vi "HitrapGUI.HTLE_TR6-LowerPart.vi"() -> ()   [LabVIEW 2014, in "HitrapGUI.lvlib"]
uses:
  HitrapGUI.lvlib
  CSlibraries/GUILib/GUILib.userEventsMainType.ctl
  CSlibraries-extern/DimLVEvent/DimIndicators/DimIndicators.anyType.ctl
  CSlibraries/GUILib/GUILib.simpleNumeric.ctl
  CSlibraries/GUILib/GUILib.basicNumeric.ctl
  CSlibraries-extern/DimLVEvent/DimIndicators/DimIndicators.numericType.ctl
  CSlibraries/UtilityLib/UtilityLib.valueStatus.ctl
  CSCore/CSSystem/CoreDefs/CoreDefs.rawDataType.ctl
  CSCore/CSSystem/CoreLib/CoreLib.double 2 byte array.vi
  CSCore/CSSystem/CoreLib/CoreLib.int 2 byte array.vi
  CSlibraries/UtilityLib/UtilityLib.lvlib
  CSCore/CSSystem/CSSystemLib/CSSystemLib.lvlib
  CSlibraries-extern/DimLVEvent/DimIndicators/DimIndicators.lvlib
  CSCore/GUIs/GOGControllerGUI/GOGControllerGUI.lvlib
  CSlibraries/GUILib/GUILib.lvlib
  CSCore/CSSystem/CoreLib/CoreLib.lvlib
  CSlibraries-extern/DimLVEvent/LVDimInterface/LVDimInterface.lvlib
panel:
  in  "TR6DK3Link":T1
  in  "MotorActivityLink-Act":T2
  in  "TR6QD3_2Ctl":T3 caption="TR6QD3_2" {"nom" step=1.0}
  in  "TR6QD3_1Ctl":T3 caption="TR6QD3_1" {"nom" step=1.0}
  in  "TR6DK3Ctl":T5 caption="TR6DK3" {"Progress Slide" scale=0.0..100.0; "Nom_Position" items=["Undefined", "Open", "Faraday Cup", "MCP"]}
  in  "userEventsMain 2":T6
  in  "userEventsMain":T6
  in  "MotorLink-Act":T2
  in  "TR6DK2Link":T1
  in  "TR6DK1Link":T1
  in  "TR6DK1Ctl":T5 caption="TR6DK1" {"Progress Slide" scale=0.0..100.0; "Nom_Position" items=["Undefined", "Open", "Faraday Cup", "MCP"]}
  in  "TR6DK2Ctl":T5 caption="TR6DK2" {"Progress Slide" scale=0.0..100.0; "Nom_Position" items=["Undefined", "Open", "Faraday Cup", "MCP"]}
  in  "Next":bool
  in  "Previous":bool
  in  "TR6QT1_3Ctl":T3 caption="TR6QT1_3" {"nom" step=1.0}
  in  "TR6QT1_2Ctl":T3 caption="TR6QT1_2" {"nom" step=1.0}
  in  "TR6KY3Ctl":T3 caption="TR6KY3" {"nom" step=1.0}
  in  "TR6DS2Ctl":T3 {"nom" step=1.0}
  in  "TR6KX3Ctl":T3 caption="TR6KX3" {"nom" step=1.0}
  in  "TR6QT1_1Ctl":T3 caption="TR6QT1_1" {"nom" step=1.0}
  in  "TR6QD2_2Ctl":T3 caption="TR6QD2_2" {"nom" step=1.0}
  in  "TR6QT1_3":bool=TRUE
  in  "TR6QT1_2":bool=TRUE
  in  "TR6QT1_1":bool=TRUE
  in  "TR6QD2_2":bool=TRUE
  in  "TR6KY3":bool=TRUE
  in  "TR6QD2_1Ctl":T3 caption="TR6QD2_1" {"nom" step=1.0}
  in  "TR6QD2_1":bool=TRUE
  in  "TR6DS2":bool=TRUE
  in  "TR5KX4":bool=TRUE
  in  "TR6MU1":bool=TRUE
  in  "TR6KY2":bool=TRUE
  in  "TR6KX2":bool=TRUE
  in  "TR6MU1Ctl":T3 caption="TR6MU1 - Field(mT)" {"nom" step=1.0}
  in  "TR6KY2Ctl":T3 caption="TR6KY2" {"nom" step=1.0}
  in  "TR6KX2Ctl":T3 caption="TR6KX2" {"nom" step=1.0}
  in  "TR6DS1":bool=TRUE
  in  "TR6DS1Ctl":T3 {"nom" step=1.0}
  in  "TR6QD1_2Ctl":T3 caption="TR6QD1_2" {"nom" step=1.0}
  in  "TR6QD1_1Ctl":T3 caption="TR6QD1_1" {"nom" step=1.0}
  in  "TR6QD1_2":bool=TRUE
  in  "TR6QD1_1":bool=TRUE
  in  "TR6KY1":bool=TRUE
  in  "TR6KY1Ctl":T3 caption="TR6KY1" {"nom" step=1.0}
  in  "TR6KX1Ctl":T3 caption="TR6KX1" {"nom" step=1.0}
  in  "TR6KX1":bool=TRUE
  in  "TR6ME1Ctl":T3 caption="TR6ME1" {"nom" step=1.0}
  in  "TR6ME1":bool=TRUE
  out "subSystem1State":string
  in  "subSystem1":bool
  out "subSystem1StateQuality":string
  in  "subControllersIgnoredDIM":T2
  in  "iniData":string
  in  "stop":bool
  in  "dummy":bool
  in  "parentSystem":bool
  in  "userEvent":refnum<user-event>
  # "TR6-LowerPart"
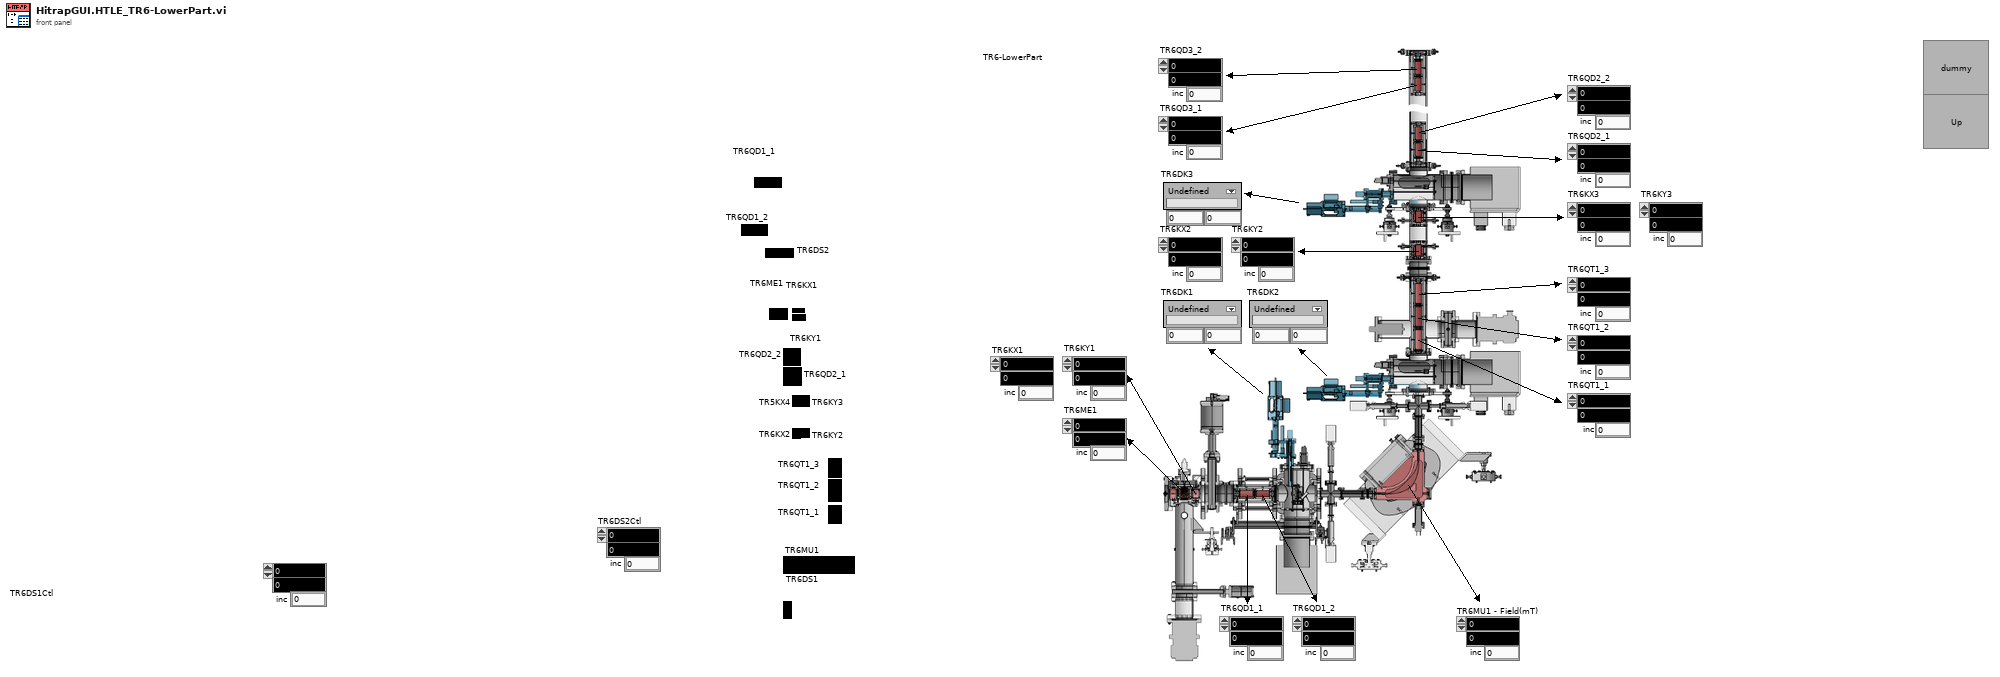
[diagram p1: front panel]
types:
  T1 = typedef "DimIndicators.lvlib/DimIndicators.numericType.ctl" = cluster{"data":dbl, "no link":bool, "quality":i32, "timeStamp":dbl}
  T2 = typedef "DimIndicators.lvlib/DimIndicators.anyType.ctl" = cluster{"data":string, "no link":bool, "quality":i32, "timeStamp":dbl}
  T3 = typedef "GUILib.lvlib/GUILib.simpleNumeric.ctl" = cluster{"nom":T4, "act":dbl, "inc":dbl}
  T4 = typedef "GUILib.lvlib/GUILib.basicNumeric.ctl" = dbl
  T5 = cluster{"Nom_Position":u8, "Progress Slide":u8, "TR6DK2Act":dbl, "TR6DK2Nom":dbl}
  T6 = typedef "GUILib.lvlib/GUILib.userEventsMainType.ctl" = cluster{"data":string, "dataType":i32}
  T7 = enum16{"Idle", "StartMotorActivity", "NewMotorDIM", "StopMotorActivity", "Stop"}
  T8 = typedef "UtilityLib.lvlib/UtilityLib.valueStatus.ctl" = enum16{"no info available", "stand by/off", "on", "warning", "alarm/malfunction", "not implemented", "user action required", "important information", "system default", "control default", "indicator default", "button default"}
  T9 = typedef "CoreDefs.rawDataType.ctl" = i8[]
  T10 = enum8{"Enabled", "Disabled", "Disabled and Grayed Out"}
  T11 = typedef "lveventtype.ctl" = enum32{"Null", "Timeout", "Annotation Menu Selection", "Annotation Menu Selection?", "App Instance Close", "App Instance Close?", "Autoscale Range Change", "Bookmark Info Change", "Cell Edit", "Cell Edit?", "Cursor Grab", "Cursor Grab?", "Cursor Menu Selection", "Cursor Menu Selection?", "Cursor Move", "Cursor Release", "Data Change", "Direction Change", "Display State Change", "Drag Ended", "Drag Enter", "Drag Leave", "Drag Over", "Drag Source Update", "Drag Starting", "Drag Starting?", "Drop", "Exec State Change", "Key Down", "Key Down?", "Key Repeat", "Key Repeat?", "Key Up", "Listbox Double Click", "Menu Activation?", "Menu Selection (App)", "Menu Selection? (App)", "Menu Selection (User)", "Mouse Down", "Mouse Down?", "Mouse Enter", "Mouse Leave", "Mouse Move", "Mouse Up", "Mouse Wheel", "NI Security User Change (App)", "Pane Size", "Panel Close", "Panel Close?", "Panel Resize", "Plot Attribute Change", "Scale Range Change", "Shortcut Menu Activation?", "Shortcut Menu Selection (App)", "Shortcut Menu Selection? (App)", "Shortcut Menu Selection (User)", "Tree Double Click", "Tree Drag", "Tree Drag?", "Tree Drop", "Tree Drop?", "Tree Item Close", "Tree Item Close?", "Tree Item Open", "Tree Item Open?", "User Event", "Value Change"}
  T12 = cluster{"TR6DK2Ctl":refnum<vi>, "byteArray out":T9}
  T13 = typedef "HitrapGUI.lvlib/HitrapGUI.i attribute.ctl" = cluster{"SVs":refnum<k21>[], "DSCIntProc":string, "MotorActivityID":i32}
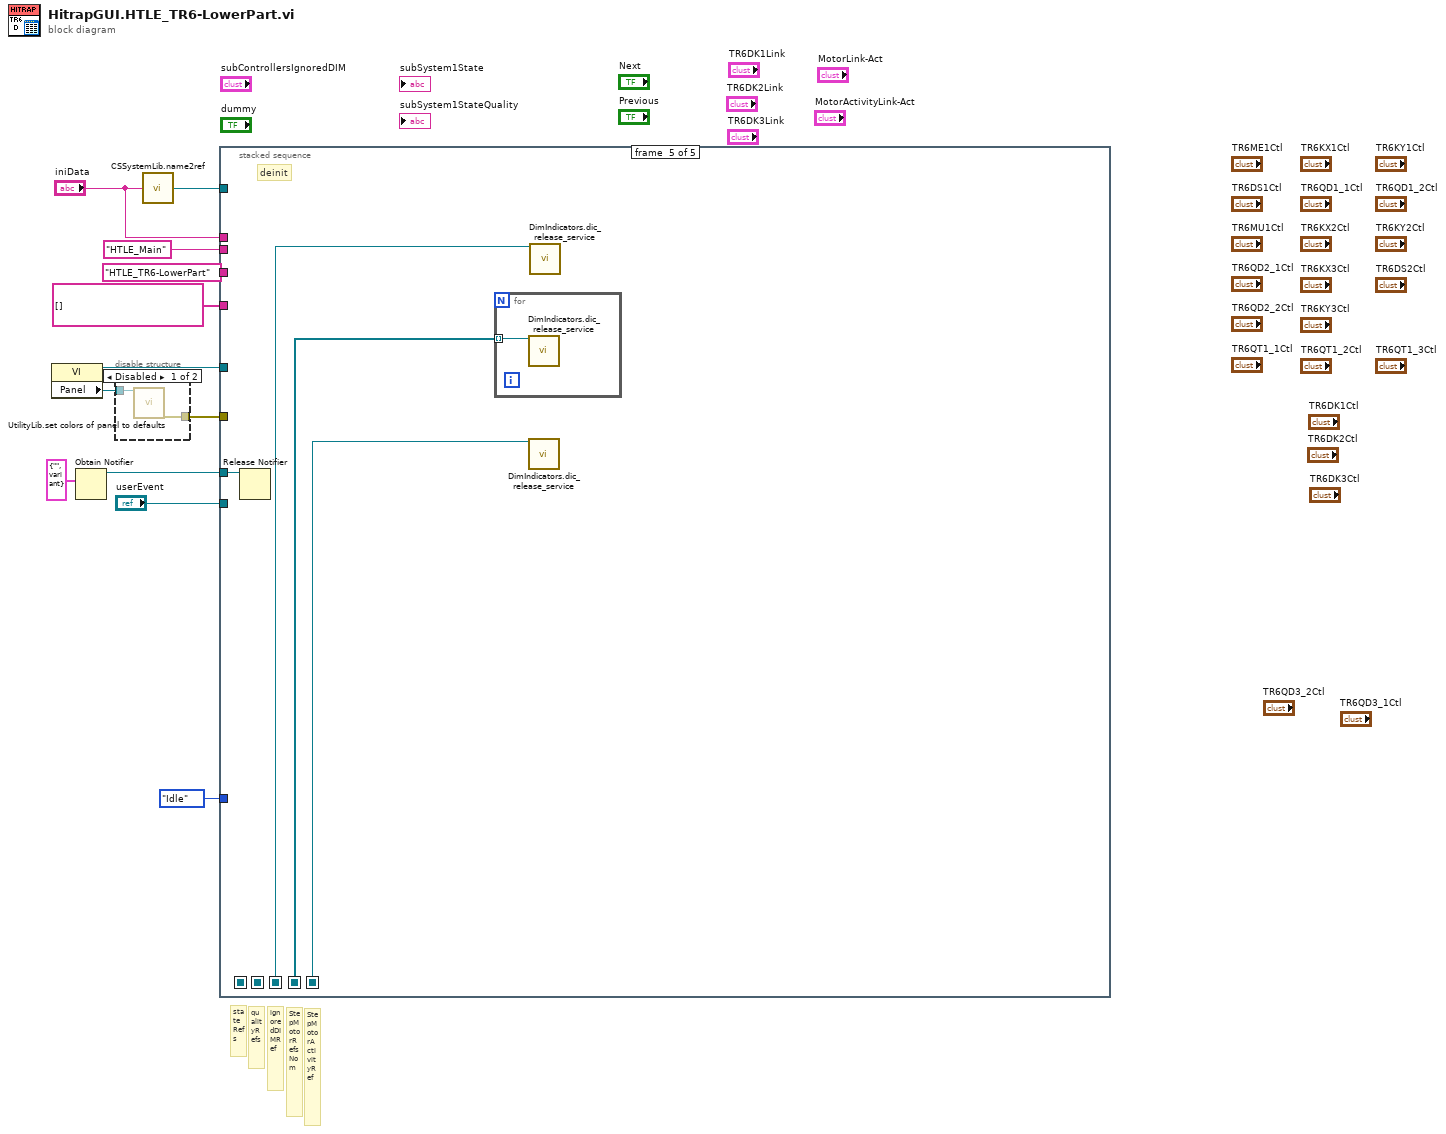
[diagram p0: block diagram]
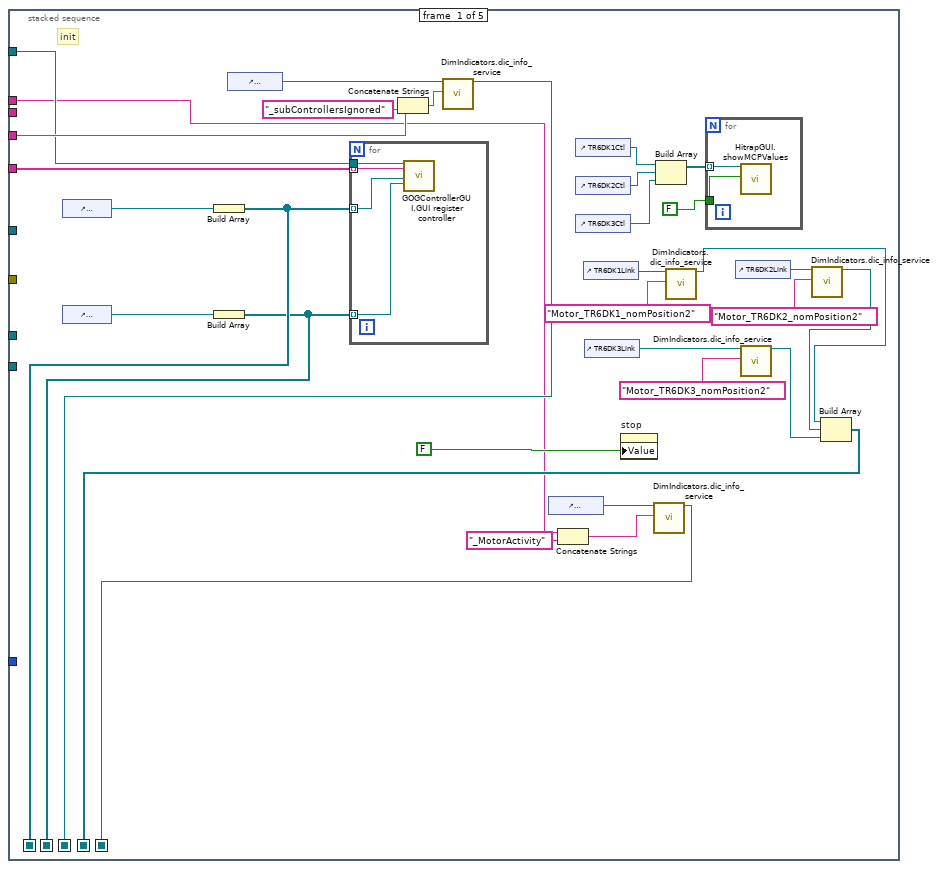
[diagram p3: hidden frame]
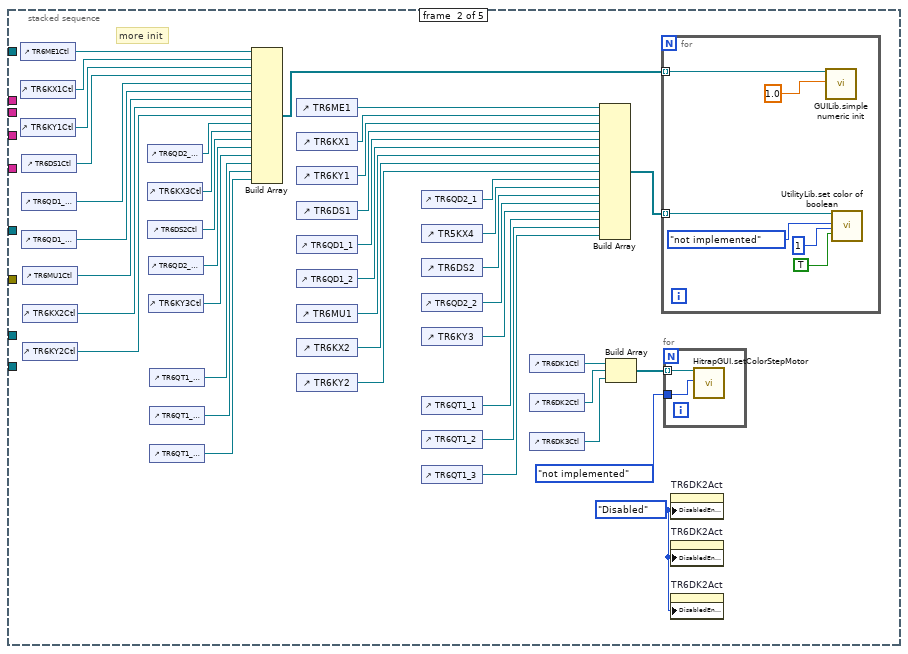
[diagram p4: hidden frame]
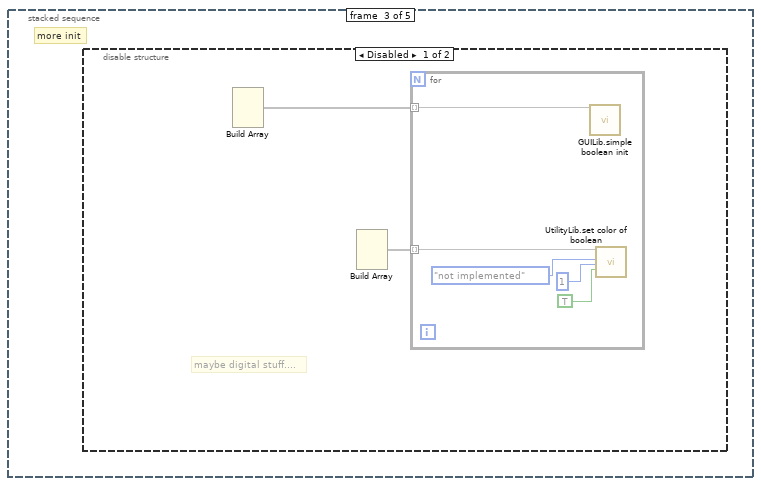
[diagram p5: hidden frame]
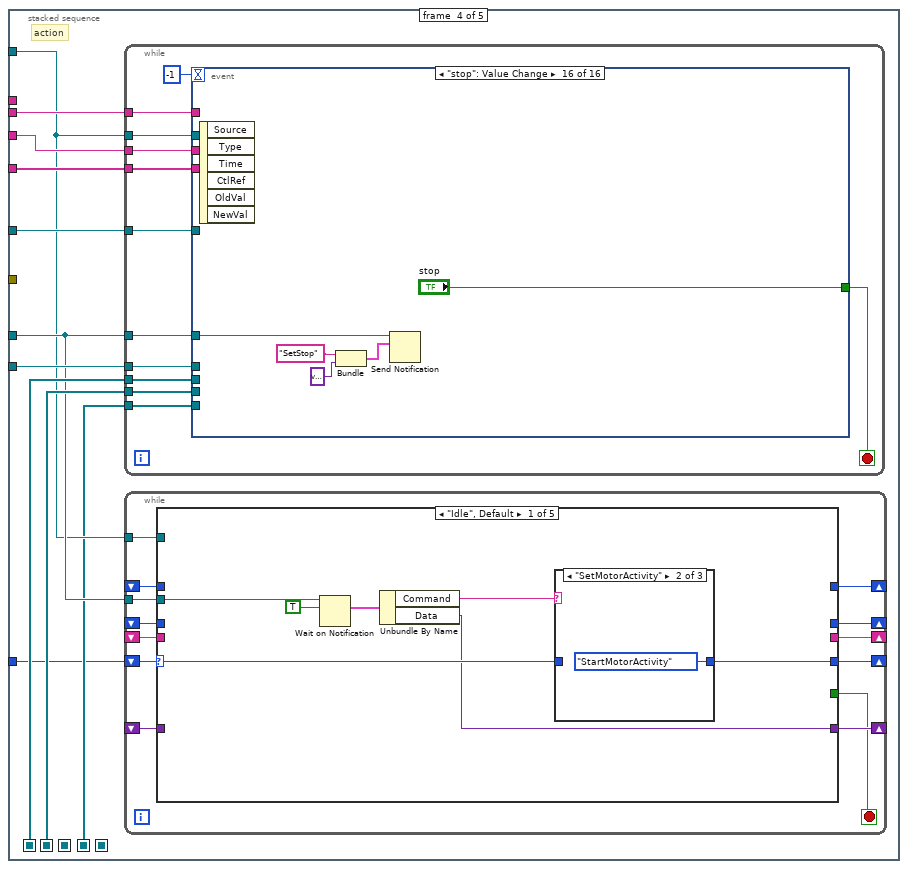
[diagram p7: hidden frame]
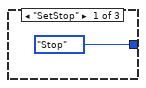
[diagram p8: hidden frame]
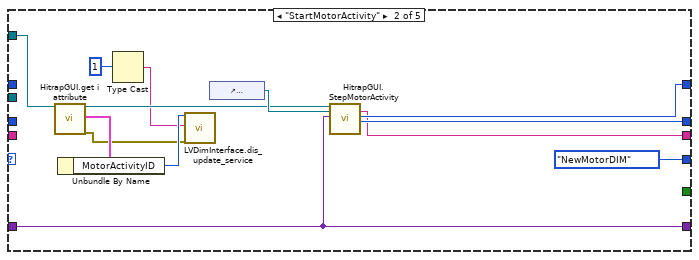
[diagram p10: hidden frame]
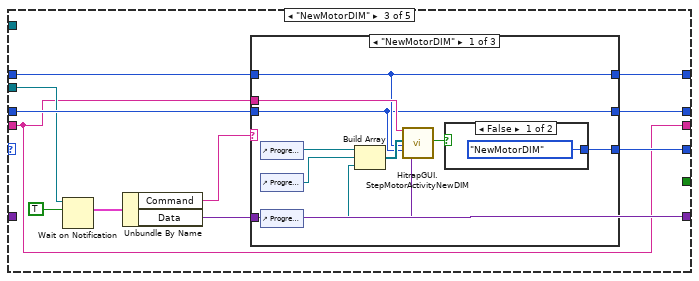
[diagram p11: hidden frame]
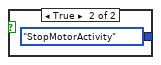
[diagram p12: hidden frame]
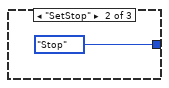
[diagram p13: hidden frame]
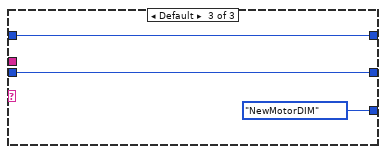
[diagram p14: hidden frame]
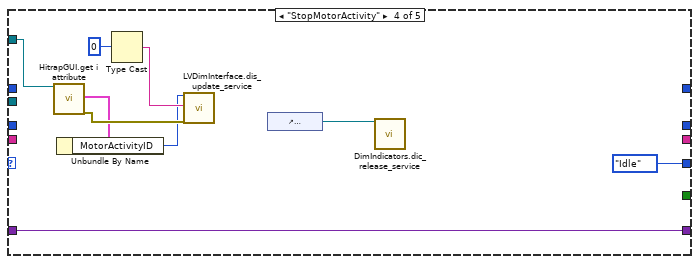
[diagram p15: hidden frame]
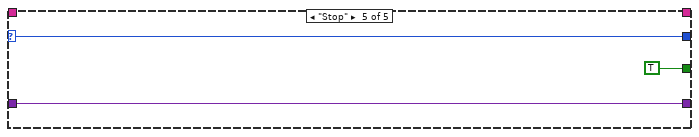
[diagram p16: hidden frame]
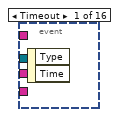
[diagram p17: hidden frame]
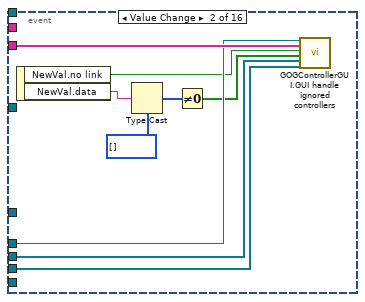
[diagram p18: hidden frame]
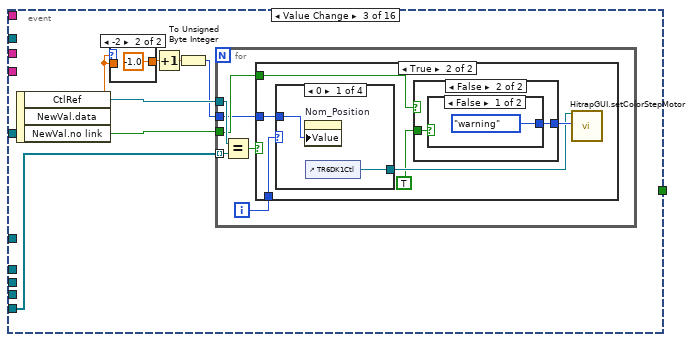
[diagram p19: hidden frame]
diagram:
  # "StepMotorActivityRef"
  # "StepMotorRefsNom"
  # "qualityRefs"
  # "ignoredDIMRef"
  # "stateRefs"
  n1 = property class="VI"() -> (reference out=w10:refnum<vi>, "Panel"=w11:refnum<vi>)  [unwired: 2 in, 1 out]
  n2 = Obtain Notifier(notification data type=cluster{"Command":string, "Data":variant} {"Command"="", "Data"=variant} ("EventData")) -> (notifier out=w4:refnum<notifier>)  [unwired: 3 in, 2 out]
  n3 = disable-structure shown="Disabled" {
    disable-tunnel: w11 -> [w14 _]
    disable-tunnel: [w13 _] -> w9
    frame Disabled {
      n4 = call "UtilityLib.set colors of panel to defaults.vi"("Front Panel"=w14) -> ("error out"=w13:errorcluster)  [unwired: 18 in]
    }
    frame Enabled {
    }
  }
  n5 = call "CSSystemLib.name2ref.vi"("name"="iniData") -> ("obj refnum"=w6:refnum<vi>)
  n6 = stacked-sequence {
    seq-local: [w36 _ _ _ _] -> [_ _ _ _ w344]
    seq-local: [w37 _ _ _ _] -> [_ _ _ w127 _]
    seq-local: [w35 _ _ _ _] -> [_ _ _ w126 _]
    seq-local: [w26 _ _ _ _] -> [_ _ _ w121 w343]
    seq-local: [w19 _ _ _ _] -> [_ _ _ _ w341]
    tunnel: "userEvent" -> [_ _ _ w130 _]
    tunnel: w10 -> [_ _ _ w129 _]
    tunnel: w9 -> [_ _ _ _ _]
    tunnel: "HTLE_TR6-LowerPart" -> [w42 _ _ w125 _]
    tunnel: string[] [] -> [w41 _ _ w128 _]
    tunnel: w6 -> [w40 _ _ w122 _]
    tunnel: "HTLE_Main" -> [_ _ _ w124 _]
    tunnel: w4 -> [_ _ _ w123 w342]
    tunnel: T7."Idle" -> [_ _ _ w120 _]
    tunnel: "iniData" -> [w21 _ _ _ _]
    frame #0 {
      # "init"
      n7 = control-ref of="dummySubSystemState"() -> (w39:refnum<vi>)
      n8 = control-ref of="dummySubSystemStateQuality"() -> (w38:refnum<vi>)
      n9 = Build Array(w39) -> (w37:refnum<vi>[])
      n10 = Build Array(w38) -> (w35:refnum<vi>[])
      n11 = control-ref of="subControllersIgnoredDIM"() -> (w43:refnum<vi>)
      n12 = for {
        tunnel: w37 -> [w52] mode=indexing
        tunnel: w41 -> [w50] mode=indexing
        tunnel: w35 -> [w49] mode=indexing
        tunnel: w40 -> [w51]
        n13 = call "GOGControllerGUI.GUI register controller.vi"("i ref in"=w51, "controllerName"=w50, "subSystemState"=w52, "subSystemStateQuality"=w49) -> ()  [unwired: 14 in, 2 out]
      }
      n14 = Concatenate Strings(w42, "_subControllersIgnored" ("string")) -> (w45:string)
      n15 = call "DimIndicators.dic_info_service.vi"("controlRef"=w43, "serviceName"=w45) -> ("controlRef out"=w36:refnum<vi>)  [unwired: 16 in, 1 out]
      n16 = control-ref of="MotorActivityLink-Act"() -> (w23:refnum<vi>)
      n17 = Concatenate Strings(w21, "_MotorActivity" ("string")) -> (w22:string)
      n18 = control-ref of="TR6DK1Ctl"() -> (w31:refnum<vi>)
      n19 = control-ref of="TR6DK2Ctl"() -> (w34:refnum<vi>)
      n20 = control-ref of="TR6DK3Ctl"() -> (w15:refnum<vi>)
      n21 = control-ref of="TR6DK1Link"() -> (w30:refnum<vi>)
      n22 = control-ref of="TR6DK3Link"() -> (w16:refnum<vi>)
      n23 = property on="stop" class="Bool (strict)"("Value"=FALSE ("stop")) -> ()  [unwired: 2 in, 2 out]
      n24 = call "DimIndicators.dic_info_service.vi"("controlRef"=w23, "serviceName"=w22) -> ("controlRef out"=w19:refnum<vi>)  [unwired: 16 in, 1 out]
      n25 = Build Array(w31, w34, w15) -> (w33:refnum<vi>[])
      n26 = call "DimIndicators.dic_info_service.vi"("controlRef"=w30, "serviceName"="Motor_TR6DK1_nomPosition2") -> ("controlRef out"=w25:refnum<vi>)  [unwired: 16 in, 1 out]
      n27 = for {
        tunnel: w33 -> [w48] mode=indexing
        tunnel: FALSE ("Visible") -> [w47]
        n28 = call "HitrapGUI.showMCPValues.vi"("Cluster Refnum"=w48, "show"=w47) -> ()  [unwired: 16 in, 2 out]
      }
      n29 = control-ref of="TR6DK2Link"() -> (w29:refnum<vi>)
      n30 = call "DimIndicators.dic_info_service.vi"("controlRef"=w16, "serviceName"="Motor_TR6DK3_nomPosition2") -> ("controlRef out"=w17:refnum<vi>)  [unwired: 16 in, 1 out]
      n31 = call "DimIndicators.dic_info_service.vi"("controlRef"=w29, "serviceName"="Motor_TR6DK2_nomPosition2") -> ("controlRef out"=w24:refnum<vi>)  [unwired: 16 in, 1 out]
      n32 = Build Array(w25, w24, w17) -> (w26:refnum<vi>[])
    }
    frame #1 {
      w53 = T10."Disabled" ("Disabled")
      # "more init"
      n33 = control-ref of="TR6ME1Ctl"() -> (w94:refnum<vi>)
      n34 = control-ref of="TR6KX1Ctl"() -> (w93:refnum<vi>)
      n35 = control-ref of="TR6KY1Ctl"() -> (w92:refnum<vi>)
      n36 = control-ref of="TR6DS1Ctl"() -> (w87:refnum<vi>)
      n37 = control-ref of="TR6QD1_1Ctl"() -> (w86:refnum<vi>)
      n38 = control-ref of="TR6QD1_2Ctl"() -> (w85:refnum<vi>)
      n39 = control-ref of="TR6MU1Ctl"() -> (w84:refnum<vi>)
      n40 = control-ref of="TR6KX2Ctl"() -> (w83:refnum<vi>)
      n41 = control-ref of="TR6KY2Ctl"() -> (w82:refnum<vi>)
      n42 = control-ref of="TR6QD2_1Ctl"() -> (w81:refnum<vi>)
      n43 = control-ref of="TR6KX3Ctl"() -> (w80:refnum<vi>)
      n44 = control-ref of="TR6DS2Ctl"() -> (w79:refnum<vi>)
      n45 = control-ref of="TR6QD2_2Ctl"() -> (w78:refnum<vi>)
      n46 = control-ref of="TR6KY3Ctl"() -> (w77:refnum<vi>)
      n47 = control-ref of="TR6QT1_1Ctl"() -> (w76:refnum<vi>)
      n48 = control-ref of="TR6QT1_2Ctl"() -> (w75:refnum<vi>)
      n49 = control-ref of="TR6QT1_3Ctl"() -> (w74:refnum<vi>)
      n50 = Build Array(w94, w93, w92, w87, w86, w85, w84, w83, w82, w81, w80, w79, w78, w77, w76, w75, w74) -> (w91:refnum<vi>[])
      n51 = control-ref of="TR6ME1"() -> (w90:refnum<vi>)
      n52 = control-ref of="TR6KX1"() -> (w89:refnum<vi>)
      n53 = control-ref of="TR6KY1"() -> (w73:refnum<vi>)
      n54 = control-ref of="TR6DS1"() -> (w72:refnum<vi>)
      n55 = control-ref of="TR6QD1_1"() -> (w71:refnum<vi>)
      n56 = control-ref of="TR6QD1_2"() -> (w70:refnum<vi>)
      n57 = control-ref of="TR6MU1"() -> (w69:refnum<vi>)
      n58 = control-ref of="TR6KX2"() -> (w68:refnum<vi>)
      n59 = control-ref of="TR6KY2"() -> (w67:refnum<vi>)
      n60 = control-ref of="TR6QD2_1"() -> (w66:refnum<vi>)
      n61 = control-ref of="TR5KX4"() -> (w65:refnum<vi>)
      n62 = control-ref of="TR6DS2"() -> (w64:refnum<vi>)
      n63 = control-ref of="TR6QD2_2"() -> (w63:refnum<vi>)
      n64 = control-ref of="TR6KY3"() -> (w62:refnum<vi>)
      n65 = control-ref of="TR6QT1_1"() -> (w61:refnum<vi>)
      n66 = control-ref of="TR6QT1_2"() -> (w60:refnum<vi>)
      n67 = control-ref of="TR6QT1_3"() -> (w59:refnum<vi>)
      n68 = control-ref of="TR6DK1Ctl"() -> (w55:refnum<vi>)
      n69 = control-ref of="TR6DK2Ctl"() -> (w56:refnum<vi>)
      n70 = control-ref of="TR6DK3Ctl"() -> (w54:refnum<vi>)
      n71 = Build Array(w90, w89, w73, w72, w71, w70, w69, w68, w67, w66, w65, w64, w63, w62, w61, w60, w59) -> (w88:refnum<vi>[])
      n72 = Build Array(w55, w56, w54) -> (w58:refnum<vi>[])
      n73 = for {
        tunnel: w91 -> [w102] mode=indexing
        tunnel: w88 -> [w98] mode=indexing
        n74 = call "GUILib.simple numeric init.vi"("ctlRef"=w102, "increment"=1.0) -> ()  [unwired: 16 in, 2 out]
        n75 = call "UtilityLib.set color of boolean.vi"("button"=w98, "valueStatus"=UtilityLib.valueStatus."not implemented", "nOfPair (0)"=1, "setTRUEColor (FALSE)"=TRUE) -> ()  [unwired: 15 in, 1 out]
      }
      n76 = for {
        tunnel: w58 -> [w96] mode=indexing
        tunnel: UtilityLib.valueStatus."not implemented" ("State") -> [w95]
        n77 = call "HitrapGUI.setColorStepMotor.vi"("Cluster Refnum"=w96, "State"=w95) -> ()  [unwired: 16 in, 2 out]
      }
      n78 = property on="TR6DK2Act" class="DigNum (strict)"("DisabledEnum"=w53) -> ()  [unwired: 2 in, 2 out]
      n79 = property on="TR6DK2Act" class="DigNum (strict)"("DisabledEnum"=w53) -> ()  [unwired: 2 in, 2 out]
      n80 = property on="TR6DK2Act" class="DigNum (strict)"("DisabledEnum"=w53) -> ()  [unwired: 2 in, 2 out]
    }
    frame #2 {
      # "more init"
      n81 = disable-structure shown="Disabled" {
        frame Disabled {
          # "maybe digital stuff...."
          n82 = Build Array() -> (w109:void[], w114:dbl, w113:dbl, w112:dbl, w111:dbl, w110:dbl)
          n83 = Build Array() -> (w103:void[], w108:dbl, w107:dbl, w106:dbl, w105:dbl, w104:dbl)
          n84 = for {
            tunnel: w109 -> [w119] mode=indexing
            tunnel: w103 -> [w115] mode=indexing
            n85 = call "GUILib.simple boolean init.vi"("ctlRef"=w119) -> ()  [unwired: 17 in, 2 out]
            n86 = call "UtilityLib.set color of boolean.vi"("button"=w115, "valueStatus"=UtilityLib.valueStatus."not implemented", "nOfPair (0)"=1, "setTRUEColor (FALSE)"=TRUE) -> ()  [unwired: 15 in, 1 out]
          }
        }
        frame Enabled {
        }
      }
    }
    frame #3 {
      # "action"
      n87 = while {
        tunnel: w130 -> [w217]
        tunnel: w129 -> [w215]
        tunnel: w128 -> [w213]
        tunnel: w127 -> [w212]
        tunnel: w126 -> [w211]
        tunnel: w122 -> [w210]
        tunnel: w125 -> [w209]
        tunnel: w124 -> [w208]
        tunnel: w121 -> [w207]
        tunnel: w123 -> [w206]
        stop <- w214 stop-if-true
        n88 = event shown="[15] \"stop\": Value Change" {
          selector: _ -> [_ _ _ _ _ _ _ _ _ _ _ _ _ _ _ _]
          dyn-events: _ -> [_ _ _ _ _ _ _ _ _ _ _ _ _ _ _ _]
          timeout: -1 -> [_ _ _ _ _ _ _ _ _ _ _ _ _ _ _ _]
          tunnel: w217 -> [_ w222 _ _ _ w269 _ w276 _ w286 w294 _ _ w327 w332 _]
          tunnel: w215 -> [_ _ _ _ _ _ _ _ _ _ _ _ _ _ _ _]
          tunnel: [_ _ _ _ _ _ _ _ _ _ _ _ _ _ _ "stop"] -> w214
          tunnel: w213 -> [_ w223 _ _ _ w265 _ _ _ _ _ _ _ _ _ _]
          tunnel: w212 -> [_ w219 _ _ _ _ _ _ _ _ _ _ _ _ _ _]
          tunnel: w211 -> [_ w218 _ _ _ _ _ _ _ _ _ _ _ _ _ _]
          tunnel: w210 -> [_ _ _ _ w262 _ _ _ _ w290 _ _ _ _ _ _]
          tunnel: w209 -> [_ _ _ _ w260 _ _ w275 _ w284 _ _ _ _ _ _]
          tunnel: w208 -> [_ _ _ _ _ w264 _ _ _ _ _ _ _ _ _ _]
          tunnel: w207 -> [_ _ w233 _ _ _ _ _ _ _ _ _ _ _ _ _]
          tunnel: w206 -> [_ _ _ _ _ _ _ _ _ _ w291 w316 _ _ _ w339]
          event Timeout {
            n89 = event-data() -> ()  [unwired: 1 in, 2 out]
          }
          event Value Change {
            n90 = event-data() -> ("NewVal.no link"=w221:bool, "NewVal.data"=w224:string)  [unwired: 1 in]
            n91 = Type Cast(type=T9 [] ("Array"), x=w224) -> (*(type *) &x=w226:T9)
            n92 = Not Equal To 0?(x=w226) -> (x != 0?=w220:bool[])
            n93 = call "GOGControllerGUI.GUI handle ignored controllers.vi"("userEvent"=w222, "controllerNames"=w223, "NOLINK"=w221, "controllersIgnored"=w220, "stateRefs"=w219, "qualityRefs"=w218) -> ()  [unwired: 14 in]
          }
          event Value Change {
            n94 = event-data() -> ("CtlRef"=w232:refnum<vi>, "NewVal.data"=w230:dbl, "NewVal.no link"=w231:bool)  [unwired: 1 in]
            n95 = case shown="-2" w230 {
              tunnel: [w234 -1.0] -> w229
              tunnel: w230 -> [w234 _]
              frame 0, Default {
              }
              frame -2 {
              }
            }
            n96 = Increment(x=w229) -> (x+1=w228:dbl)
            n97 = To Unsigned Byte Integer(number=w228) -> (unsigned 8bit integer=w227:u8)
            n98 = for {
              tunnel: w233 -> [w237] mode=indexing
              tunnel: w232 -> [w241]
              tunnel: w231 -> [w238]
              tunnel: w227 -> [w236]
              i -> [w239]
              n99 = Equal?(x=w241, y=w237) -> (x = y?=w240:bool)
              n100 = case shown="True" w240 {
                tunnel: w236 -> [_ w246]
                tunnel: w239 -> [_ w247]
                tunnel: w238 -> [_ w244]
                frame False {
                }
                frame True {
                  n101 = case shown="0" w247 {
                    tunnel: w246 -> [w254 w256 w258 _]
                    tunnel: [w253 w255 w257 _] -> w243
                    frame 0 {
                      n102 = property on="Nom_Position" class="Ring (strict)"("Value"=w254) -> ()  [unwired: 2 in, 2 out]
                      n103 = control-ref of="TR6DK1Ctl"() -> (w253:refnum<vi>)
                    }
                    frame 1 {
                      n104 = property on="Nom_Position" class="Ring (strict)"("Value"=w256) -> ()  [unwired: 2 in, 2 out]
                      n105 = control-ref of="TR6DK2Ctl"() -> (w255:refnum<vi>)
                    }
                    frame 2 {
                      n106 = property on="Nom_Position" class="Ring (strict)"("Value"=w258) -> ()  [unwired: 2 in, 2 out]
                      n107 = control-ref of="TR6DK3Ctl"() -> (w257:refnum<vi>)
                    }
                    frame Default {
                    }
                  }
                  n108 = case shown="False" w244 {
                    tunnel: [UtilityLib.valueStatus."not implemented" ("State") w250] -> w245
                    tunnel: TRUE -> [_ w249]
                    frame True {
                    }
                    frame False {
                      n109 = case shown="False" w249 {
                        tunnel: [UtilityLib.valueStatus."warning" ("State") UtilityLib.valueStatus."on" ("State")] -> w250
                        frame False {
                        }
                        frame True {
                        }
                      }
                    }
                  }
                  n110 = call "HitrapGUI.setColorStepMotor.vi"("Cluster Refnum"=w243, "State"=w245) -> ()  [unwired: 16 in, 2 out]
                }
              }
            }
          }
          event Panel Close? {
            n111 = event-data() -> ()  [unwired: 1 in, 4 out]
            n112 = event-data("Discard?"=TRUE) -> ()  [unwired: 1 in, 1 out]
          }
          event "TR6ME1", "TR6DS1", "TR6MU1", "TR6QD2_1", "TR6QD2_2", "TR6QT1_1", "TR6KX1", "TR6QD1_1", "TR6KX2", "TR5KX4", "TR6KY3", "TR6QT1_2", "TR6KY1", "TR6QD1_2", "TR6KY2", "TR6DS2", "TR6QT1_3": Value Change {
            n113 = event-data() -> ("CtlRef"=w261:refnum<vi>)  [unwired: 1 in]
            n114 = call "GOGControllerGUI.GUI open front panel.vi"("i ref in"=w262, "elementRef"=w261, "controller"=w260) -> ()  [unwired: 15 in, 2 out]
          }
          event "subSystem1", "parentSystem": Value Change {
            n115 = event-data() -> ("CtlRef"=w267:refnum<vi>)  [unwired: 1 in]
            n116 = control-ref of="parentSystem"() -> (w266:refnum<vi>)
            n117 = control-ref of="subSystem1"() -> (w270:refnum<vi>)
            n118 = Build Array (concatenate)(w264, w265) -> (w263:string[])
            n119 = Build Array(w266, w270) -> (w268:refnum<vi>[])
            n120 = call "GOGControllerGUI.GUI set selected subcontroller.vi"("userEvent"=w269, "controllerNames"=w263, "controllerRefs"=w268, "controllerRef"=w267) -> ()  [unwired: 16 in]
          }
          event Value Change {
            n121 = event-data() -> ("CtlRef"=w272:refnum<vi>, "NewVal"=w271:dbl)  [unwired: 1 in]
            n122 = call "GUILib.simple numeric change increment.vi"("ctlRef"=w272, "increment"=w271) -> ()  [unwired: 16 in, 2 out]
          }
          event Mouse Enter; Mouse Leave {
            n123 = event-data() -> ("CtlRef"=w274:refnum<vi>, "Type"=w273:T11)  [unwired: 1 in]
            n124 = case shown="\"Mouse Enter\"" w273 {
              tunnel: [TRUE _] -> w277
              frame "Mouse Enter" {
              }
              frame Default {
              }
            }
            n125 = call "GUILib.simple numeric show increment.vi"("ctlRef"=w274, "show"=w277) -> ("error out"=w278:errorcluster)  [unwired: 16 in, 1 out]
            n126 = call "GOGControllerGUI.GUI set error.vi"("userEvent"=w276, "controller"=w275, "GUIError"=w278) -> ()  [unwired: 16 in, 1 out]
          }
          event "TR6DK2Ctl", "TR6DK1Ctl", "TR6DK3Ctl": Mouse Enter; "TR6DK1Ctl", "TR6DK2Ctl", "TR6DK3Ctl": Mouse Leave {
            n127 = event-data() -> ("CtlRef"=w281:refnum<vi>, "Type"=w282:T11)  [unwired: 1 in]
            n128 = case shown="\"Mouse Enter\"" w282 {
              tunnel: [TRUE _] -> w280
              frame "Mouse Enter" {
              }
              frame Default {
              }
            }
            n129 = call "HitrapGUI.showMCPValues.vi"("Cluster Refnum"=w281, "show"=w280) -> ()  [unwired: 16 in, 2 out]
          }
          event Value Change {
            n130 = event-data() -> ("CtlRef"=w289:refnum<vi>, "NewVal"=w288:T4)  [unwired: 1 in]
            n131 = call-poly "CoreLib.data 2 byte array.vi"("f64"=w288) -> ("byteArray out"=w287:T9)  [unwired: 18 in]
            n132 = call "GOGControllerGUI.GUI set nominal value.vi"("i ref in"=w290, "nominalRef"=w289, "nominalData"=w287, "controller"=w284) -> ("error out"=w285:errorcluster)  [unwired: 14 in, 1 out]
            n133 = call "GOGControllerGUI.GUI set error.vi"("userEvent"=w286, "controller"=w284, "GUIError"=w285) -> ()  [unwired: 16 in, 1 out]
          }
          event "TR6DK2Ctl.Nom_Position", "TR6DK1Ctl.Nom_Position", "TR6DK3Ctl.Nom_Position": Value Change {
            n134 = event-data() -> ("CtlRef"=w295:refnum<vi>, "NewVal"=w292:u8)  [unwired: 1 in, 1 out]
            n135 = Greater Than 0?(x=w292) -> (x > 0?=w293:bool)
            n136 = case shown="False" w293 {
              tunnel: w295 -> [_ w308]
              tunnel: w294 -> [_ _]
              tunnel: w292 -> [_ w309]
              tunnel: w291 -> [_ w307]
              frame False {
              }
              frame True {
                n137 = Decrement(x=w309) -> (x-1=w300:u8)
                n138 = property class="Ring (strict)"(reference=w308) -> ("Owner"=w298:refnum<vi>)  [unwired: 1 in, 2 out]
                n139 = call-poly "CoreLib.data 2 byte array.vi"("i32"=0) -> ("byteArray out"=w302:T9)  [unwired: 18 in]
                n140 = call-poly "CoreLib.data 2 byte array.vi"("byteArray"=w302, "i32"=w300) -> ("byteArray out"=w299:T9)  [unwired: 17 in]
                n141 = control-ref of="TR6DK2Ctl"() -> (w297:refnum<vi>)
                n142 = To More Specific Class(target class=w297, reference=w298) -> (specific class reference=w296:refnum<vi>)  [unwired: 1 in, 1 out]
                n143 = Bundle("TR6DK2Ctl"=w296, "byteArray out"=w299) -> (w303:T12)  [unwired: 1 in]
                n144 = To Variant(anything=w303) -> (Variant=w304:variant)
                n145 = Bundle("SetMotorActivity", "Variant"=w304) -> (w306:cluster{string, "Variant":variant})  [unwired: 1 in]
                n146 = Send Notification(notification=w306, notifier=w307) -> ()  [unwired: 1 in, 2 out]
              }
            }
          }
          event Value Change {
            w311 = 0.0
            n147 = event-data() -> ("OldVal"=w314:string, "NewVal"=w312:string)  [unwired: 1 in, 1 out]
            n148 = Type Cast(type=w311, x=w312) -> (*(type *) &x=w310:dbl)
            n149 = Type Cast(type=w311, x=w314) -> (*(type *) &x=w313:dbl)
            n150 = Bundle(w313, w310) -> (w315:cluster{dbl, dbl})  [unwired: 1 in]
            n151 = To Variant(anything=w315) -> (Variant=w317:variant)
            n152 = Bundle("NewMotorDIM", "Variant"=w317) -> (w319:cluster{string, "Variant":variant})  [unwired: 1 in]
            n153 = Send Notification(notification=w319, notifier=w316) -> ()  [unwired: 1 in, 2 out]
          }
          event Value Change {
            n154 = event-data() -> ("NewVal"=w323:string)  [unwired: 1 in, 2 out]
            n155 = Type Cast(type=i16 0 ("x"), x=w323) -> (*(type *) &x=w321:i16)
            n156 = case shown="1" w321 {
              tunnel: [T10."Enabled" ("Disabled") T10."Disabled and Grayed Out" ("Disabled")] -> w320
              frame 0, Default {
              }
              frame 1 {
              }
            }
            n157 = property on="TR6DK1Ctl" class="Clust (strict)"("DisabledEnum"=w320) -> ()  [unwired: 2 in, 2 out]
            n158 = property on="TR6DK2Ctl" class="Clust (strict)"("DisabledEnum"=w320) -> ()  [unwired: 2 in, 2 out]
            n159 = property on="TR6DK3Ctl" class="Clust (strict)"("DisabledEnum"=w320) -> ()  [unwired: 2 in, 2 out]
          }
          event "Next": Value Change {
            n160 = event-data() -> ()  [unwired: 1 in, 3 out]
            n161 = Bundle By Name(cluster="userEventsMain", "data"="HTLE_TR6-UpperPart", "dataType"=0) -> (w330:T6)
            n162 = Generate User Event(user event=w327, event data cluster=w330) -> ()  [unwired: 2 in, 2 out]
          }
          event "Previous": Value Change {
            n163 = event-data() -> ()  [unwired: 1 in, 3 out]
            n164 = Bundle By Name(cluster="userEventsMain 2", "data"="HTLE_TR6BT1", "dataType"=0) -> (w335:T6)
            n165 = Generate User Event(user event=w332, event data cluster=w335) -> ()  [unwired: 2 in, 2 out]
          }
          event "stop": Value Change {
            n166 = event-data() -> ()  [unwired: 1 in, 6 out]
            n167 = Bundle("SetStop", "Data"=variant) -> (w338:cluster{string, "Data":variant})  [unwired: 1 in]
            n168 = Send Notification(notification=w338, notifier=w339) -> ()  [unwired: 1 in, 2 out]
          }
        }
      }
      n169 = while {
        tunnel: w123 -> [w143]
        shift-right: [w142] -> _
        shift-left: _ -> [w141]
        tunnel: w122 -> [w140]
        shift-right: [w138] -> _
        shift-left: _ -> [w137]
        shift-right: [w139] -> _
        shift-left: _ -> [w136]
        shift-right: [w133] -> _
        shift-left: _ -> [w134]
        shift-right: [w131] -> _
        shift-left: w120 -> [w132]
        stop <- w135 stop-if-true
        n170 = case shown="\"Idle\", Default" w132 {
          selector: w132 -> [w147 _ _ _ w204]
          tunnel: w143 -> [w150 _ w172 _ _]
          tunnel: [w146 w164 w170 w202 w205] -> w142
          tunnel: w141 -> [_ w164 _ w202 w205]
          tunnel: w140 -> [_ w160 _ w194 _]
          tunnel: [w144 T7."NewMotorDIM" w177 T7."Idle" w204] -> w131
          tunnel: [_ w165 w167 _ _] -> w139
          tunnel: [_ w166 w168 _ _] -> w138
          tunnel: w137 -> [_ _ w176 _ _]
          tunnel: w136 -> [_ _ w175 _ _]
          tunnel: [_ _ _ _ TRUE] -> w135
          tunnel: w134 -> [_ _ w169 _ _]
          tunnel: [_ w162 w169 _ _] -> w133
          frame "Idle", Default {
            n171 = Wait on Notification(notifier=w150, ignore previous (F)=TRUE) -> (notification=w149:cluster{"Command":string, "Data":variant})  [unwired: 2 in, 3 out]
            n172 = Unbundle By Name(w149) -> ("Command"=w148:string, "Data"=w146:variant)
            n173 = case shown="\"SetMotorActivity\"" w148 {
              tunnel: w147 -> [_ _ w153]
              tunnel: [T7."Stop" T7."StartMotorActivity" w153] -> w144
              frame "SetStop" {
              }
              frame "SetMotorActivity" {
              }
              frame "Idle", Default {
              }
            }
          }
          frame "StartMotorActivity" {
            n174 = call "HitrapGUI.get i attribute.vi"("i ref in"=w160) -> ("i ref out"=w159:refnum<vi>, "i attribute"=w158:T13, "error out"=w156:errorcluster)  [unwired: 16 in]
            n175 = Unbundle By Name(w158) -> ("MotorActivityID"=w157:i32)
            n176 = Type Cast(x=i16 1) -> (*(type *) &x=w154:string)  [unwired: 1 in]
            n177 = call "LVDimInterface.dis_update_service.vi"("my_serviceID"=w157, "data"=w154, "error in (no error)"=w156) -> ()  [unwired: 14 in, 3 out]
            n178 = control-ref of="MotorLink-Act"() -> (w163:refnum<vi>)
            n179 = call "HitrapGUI.StepMotorActivity.vi"("i ref in"=w159, "DIMPositioncontrolRef"=w163, "Data"=w164) -> ("MotorName"=w162:string, "StartPosition"=w166:i32, "StopPosition"=w165:i32)  [unwired: 12 in, 2 out]
          }
          frame "NewMotorDIM" {
            n180 = Wait on Notification(notifier=w172, ignore previous (F)=TRUE) -> (notification=w173:cluster{"Command":string, "Data":variant})  [unwired: 2 in, 3 out]
            n181 = Unbundle By Name(w173) -> ("Command"=w171:string, "Data"=w170:variant)
            n182 = case shown="\"NewMotorDIM\"" w171 {
              tunnel: [w185 T7."Stop" T7."NewMotorDIM"] -> w177
              tunnel: w176 -> [w180 _ w192]
              tunnel: w175 -> [w179 _ w191]
              tunnel: w170 -> [w182 _ _]
              tunnel: w169 -> [w181 _ _]
              tunnel: [w180 _ w192] -> w168
              tunnel: [w179 _ w191] -> w167
              frame "NewMotorDIM" {
                n183 = control-ref of="Progress Slide"() -> (w186:refnum<vi>)
                n184 = control-ref of="Progress Slide"() -> (w187:refnum<vi>)
                n185 = control-ref of="Progress Slide"() -> (w178:refnum<vi>)
                n186 = Build Array(w186, w187, w178) -> (w183:refnum<vi>[])
                n187 = call "HitrapGUI.StepMotorActivityNewDIM.vi"("MotorName"=w181, "Progress Slide Array"=w183, "StartPosition"=w180, "StopPosition"=w179, "Data"=w182) -> ("Finished?"=w184:bool)  [unwired: 12 in, 2 out]
                n188 = case shown="False" w184 {
                  tunnel: [T7."NewMotorDIM" T7."StopMotorActivity"] -> w185
                  frame False {
                  }
                  frame True {
                  }
                }
              }
              frame "SetStop" {
              }
              frame Default {
              }
            }
          }
          frame "StopMotorActivity" {
            n189 = call "HitrapGUI.get i attribute.vi"("i ref in"=w194) -> ("i attribute"=w195:T13, "error out"=w197:errorcluster)  [unwired: 16 in, 1 out]
            n190 = Unbundle By Name(w195) -> ("MotorActivityID"=w196:i32)
            n191 = Type Cast(x=i16 0) -> (*(type *) &x=w199:string)  [unwired: 1 in]
            n192 = call "LVDimInterface.dis_update_service.vi"("my_serviceID"=w196, "data"=w199, "error in (no error)"=w197) -> ()  [unwired: 14 in, 3 out]
            n193 = control-ref of="MotorLink-Act"() -> (w200:refnum<vi>)
            n194 = call "DimIndicators.dic_release_service.vi"("controlRef"=w200) -> ()  [unwired: 18 in, 1 out]
          }
          frame "Stop" {
          }
        }
      }
    }
    frame #4 {
      # "deinit"
      n195 = Release Notifier(notifier=w342) -> ()  [unwired: 2 in, 3 out]
      n196 = for {
        tunnel: w343 -> [w345] mode=indexing
        n197 = call "DimIndicators.dic_release_service.vi"("controlRef"=w345) -> ()  [unwired: 18 in, 1 out]
      }
      n198 = call "DimIndicators.dic_release_service.vi"("controlRef"=w341) -> ()  [unwired: 18 in, 1 out]
      n199 = call "DimIndicators.dic_release_service.vi"("controlRef"=w344) -> ()  [unwired: 18 in, 1 out]
    }
  }
